vi "DAQ_Mic.vi"() -> ()   [LabVIEW 2020]
panel:
  in  "stop (F)":bool
  out "Waveform Graph":dynamicdata(graph)
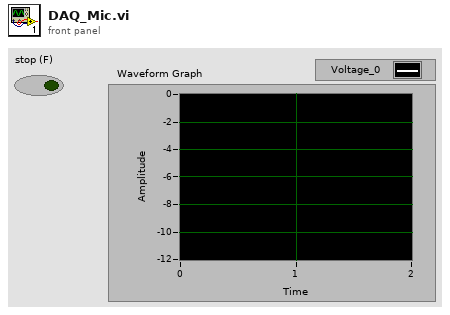
[diagram p1: front panel]
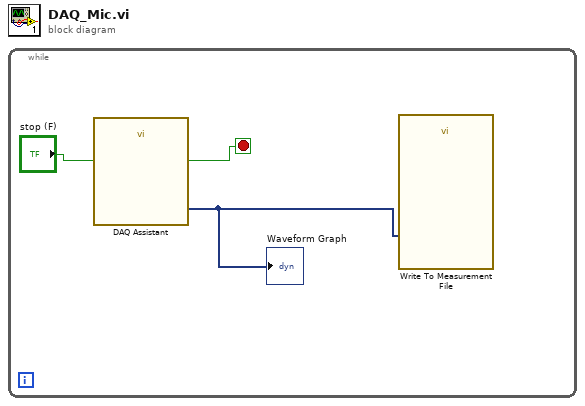
[diagram p0: block diagram]
diagram:
  n1 = while {
    stop <- w1 stop-if-true
    n2 = call "DAQ Assistant"("stop (F)"="stop (F)") -> ("data"=w2:dynamicdata, "stopped"=w1:bool)  [unwired: 15 in, 2 out]
    "Waveform Graph" <- w2
    n3 = call "Write To Measurement File"("Signals"=w2) -> ()  [unwired: 16 in, 3 out]
  }
